vi "Get column name.vi"(8 "error in (no error)":errorcluster, 11 "Column in":refnum<class "Composed Column.lvclass">) -> (0 "error out":errorcluster, 2 "Name":string, 3 "Column out":refnum<class "Composed Column.lvclass">)   [LabVIEW 2020, in "Composed Columns.lvlib" / "Composed Column.lvclass"]
uses:
  Composed Column.lvclass
  Composed Column.lvclass/Composed Column.ctl
  Basic Columns/Column Configuration/Basic Column Configuration Class/Column Configuration.lvclass
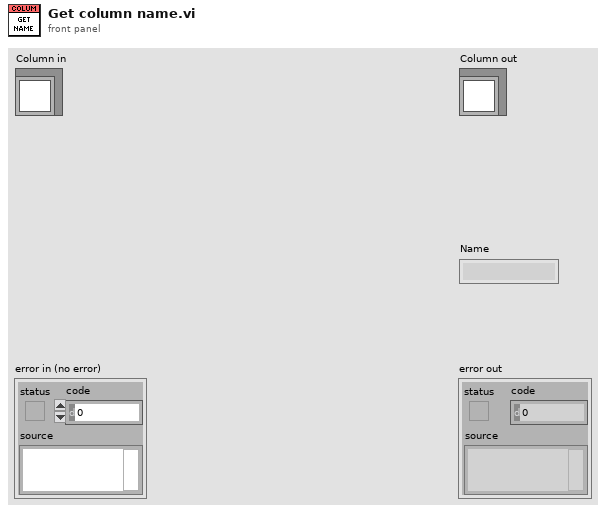
[diagram p1: front panel]
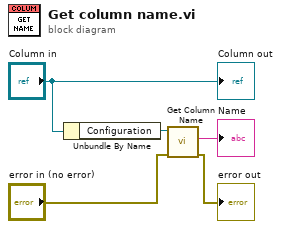
[diagram p0: block diagram]
diagram:
  n1 = Unbundle By Name("Column in") -> ("Configuration"=w5:refnum<class "Column Configuration.lvclass">)
  n2 = call-dynamic "Get Column Name.vi"("error in (no error)"="error in (no error)", "Basic Column Configuration in"=w5) -> ("error out"=→"error out":errorcluster, "Column Name"=→"Name":string)  [unwired: 7 in, 1 out]
  "Column out" <- "Column in"
